vi "ConvertGoop3ToGoop4_RemoveAlwaysCopy.vi"(8 "error in (no error)":errorcluster, 10 "BaseClasses":path[](array[path]), 11 "ViRef":refnum<vi>) -> (0 "error out":errorcluster, 3 "ViRefOut":refnum<vi>)   [LabVIEW 2020]
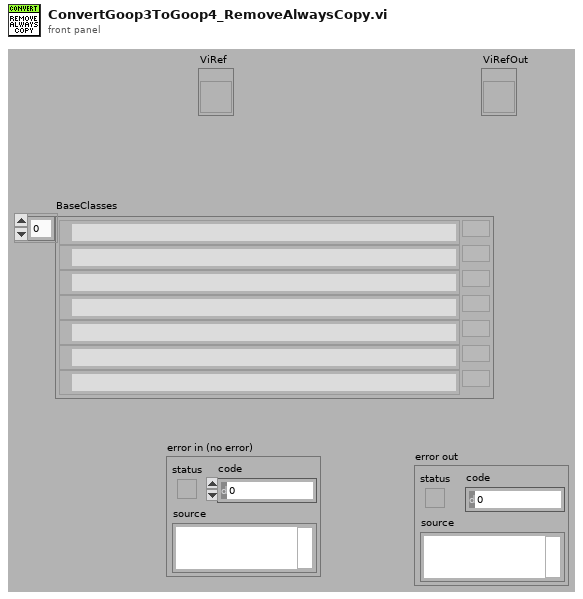
[diagram p1: front panel]
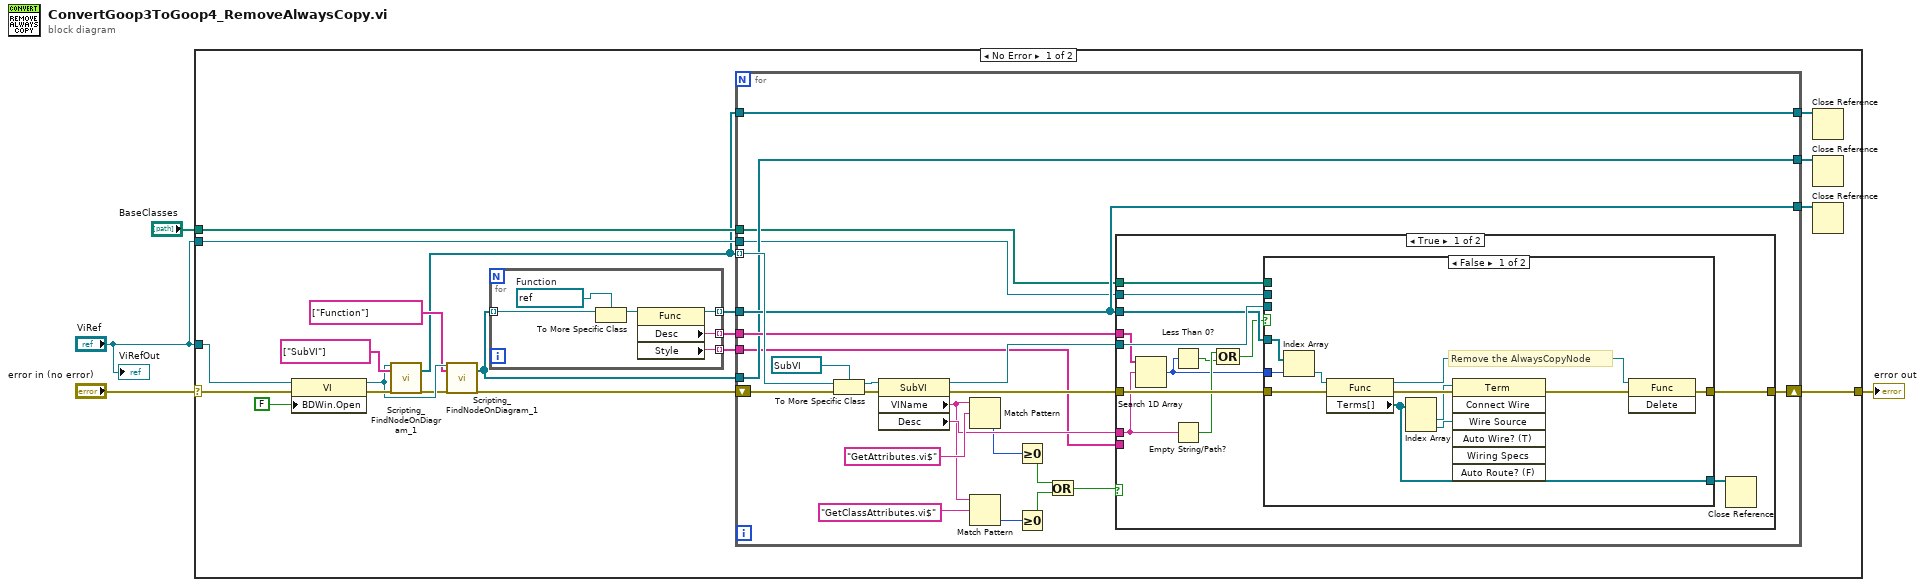
[diagram p0: block diagram]
diagram:
  n1 = case shown="No Error" "error in (no error)" {
    selector: "error in (no error)" -> [w19 w81]
    tunnel: [w22 w81] -> w4
    tunnel: "ViRef" -> [w20 _]
    tunnel: "BaseClasses" -> [w7 _]
    tunnel: "ViRef" -> [w6 _]
    frame No Error {
      n2 = property class="VI"(reference=w20, error in=w19, "BDWin.Open"=FALSE ("Front Panel Window:Open")) -> (reference out=w18:refnum<vi>, error out=w21:errorcluster)
      n3 = call "Scripting_FindNodeOnDiagram_1.vi"("ViRef(Ignored If Not Wired)"=w18, "NodeTypesToSearchFor"=string[] ["SubVI"], "error in (no error)"=w21) -> ("Nodes"=w5:refnum<vi>[], "error out"=w16:errorcluster)  [unwired: 15 in]
      n4 = call "Scripting_FindNodeOnDiagram_1.vi"("ViRef(Ignored If Not Wired)"=w18, "NodeTypesToSearchFor"=string[] ["Function"], "error in (no error)"=w16) -> ("Nodes"=w11:refnum<vi>[], "error out"=w15:errorcluster)  [unwired: 15 in]
      n5 = for {
        tunnel: w11 -> [w28] mode=indexing
        tunnel: [w27] -> w14 mode=indexing
        tunnel: [w26] -> w13 mode=indexing
        tunnel: [w25] -> w8 mode=indexing
        w29 = refnum<vi> refnum  # Function
        n6 = To More Specific Class(target class=w29, reference=w28) -> (specific class reference=w30:refnum<vi>)  [unwired: 1 in, 1 out]
        n7 = property class="Func"(reference=w30) -> (reference out=w26:refnum<vi>, "Desc"=w27:string, "Style"=w25:string)  [unwired: 1 in, 1 out]
      }
      n8 = for {
        tunnel: w5 -> [w54] mode=indexing
        shift-right: [w41] -> w22
        shift-left: w15 -> [w52]
        tunnel: w14 -> [w45]
        tunnel: w13 -> [w44]
        tunnel: [w44] -> w12
        tunnel: w11 -> [w43]
        tunnel: [w43] -> w10
        tunnel: w5 -> [w42]
        tunnel: [w42] -> w9
        tunnel: w8 -> [w40]
        tunnel: w7 -> [w39]
        tunnel: w6 -> [w38]
        n9 = To More Specific Class(target class=refnum<vi> refnum ("WhileLoop"), reference=w54, error in=w52) -> (specific class reference=w51:refnum<vi>, error out=w50:errorcluster)
        n10 = property class="SubVI"(reference=w51, error in=w50) -> (reference out=w48:refnum<vi>, error out=w47:errorcluster, "VIName"=w36:string, "Desc"=w46:string)
        n11 = Match Pattern(string=w36, regular expression="GetAttributes.vi$") -> (offset past match=w35:i32)  [unwired: 1 in, 3 out]
        n12 = Match Pattern(string=w36, regular expression="GetClassAttributes.vi$") -> (offset past match=w34:i32)  [unwired: 1 in, 3 out]
        n13 = Greater Or Equal To 0?(x=w35) -> (x >= 0?=w33:bool)
        n14 = Greater Or Equal To 0?(x=w34) -> (x >= 0?=w32:bool)
        n15 = Or(x=w33, y=w32) -> (x .or. y?=w31:bool)
        n16 = case shown="True" w31 {
          tunnel: w48 -> [w67 _]
          tunnel: w47 -> [w66 w80]
          tunnel: [w65 w80] -> w41
          tunnel: w46 -> [w60 _]
          tunnel: w45 -> [w64 _]
          tunnel: w44 -> [w63 _]
          tunnel: w40 -> [_ _]
          tunnel: w39 -> [w62 _]
          tunnel: w38 -> [w61 _]
          frame True {
            n17 = Search 1D Array(1D array=w64, element=w60) -> (index of element=w58:i32)  [unwired: 1 in]
            n18 = Less Than 0?(x=w58) -> (x < 0?=w57:bool)
            n19 = Empty String/Path?(string/path=w60) -> (empty?=w59:bool)
            n20 = Compound Arithmetic op=OR(w59, w57) -> (w56:bool)
            n21 = case shown="False" w56 {
              tunnel: w67 -> [_ _]
              tunnel: w66 -> [w76 w79]
              tunnel: [w74 w79] -> w65
              tunnel: w63 -> [w78 _]
              tunnel: w62 -> [_ _]
              tunnel: w61 -> [_ _]
              tunnel: w58 -> [w75 _]
              tunnel: [w72 _] -> w55
              frame False {
                # "Remove the AlwaysCopyNode"
                n22 = Index Array(array=w78, index=w75) -> (element=w77:refnum<vi>)
                n23 = property class="Func"(reference=w77, error in=w76) -> (reference out=w73:refnum<vi>, error out=w71:errorcluster, "Terms[]"=w72:refnum<vi>[])
                n24 = Index Array(array=w72) -> (element #1=w70:refnum<vi>, element #2=w69:refnum<vi>)  [unwired: 2 in]
                n25 = invoke class="Term" method="Connect Wire"(reference=w70, error in=w71, "Wire Source"=w69) -> (error out=w68:errorcluster)  [unwired: 4 in, 6 out]
                n26 = invoke class="Func" method="Delete"(reference=w73, error in=w68) -> (error out=w74:errorcluster)  [unwired: 1 in, 2 out]
              }
              frame True {
              }
            }
            n27 = Close Reference(reference=w55) -> ()  [unwired: 1 in, 1 out]
          }
          frame False {
          }
        }
      }
      n28 = Close Reference(reference=w9) -> ()  [unwired: 1 in, 1 out]
      n29 = Close Reference(reference=w10) -> ()  [unwired: 1 in, 1 out]
      n30 = Close Reference(reference=w12) -> ()  [unwired: 1 in, 1 out]
    }
    frame Error {
    }
  }
  "error out" <- w4
  "ViRefOut" <- "ViRef"
